vi "Promote Glue Routines.vi"(8 "error in (no error)":errorcluster, 11 "Assembly Run in":refnum<class "Assembly Run.lvclass">) -> (0 "error out":errorcluster, 3 "Assembly Run out":refnum<class "Assembly Run.lvclass">)   [LabVIEW 2021, in "Assembly Run.lvclass"]
uses:
  Assembly Run.lvclass
  Assembly Run.lvclass/Assembly Run.ctl
  Routine/Settings.ctl
  Routine/Routine Enum.ctl
  Workspace/Fixture Enum.ctl
  Workspace/Fixture.lvclass
  Routine/Routine.lvclass
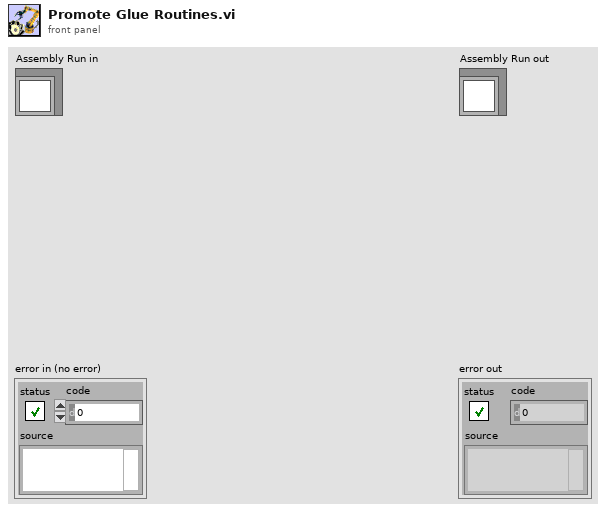
[diagram p1: front panel]
types:
  T1 = typedef "Fixture.lvclass/Fixture Enum.ctl" = enum16{"Assembly Tray", "Syringe Space", "Component", "Pick Up Tool", "Current Position"}
  T2 = typedef "Routine.lvclass/Routine Enum.ctl" = enum16{"Primary Pick Up", "Secondary Pick Up", "Put Down All", "Secure Syringe", "Release Syringe", "Dispense on Plate", "Dispense on Sensor", "Pick Up All", "Put Down Secondary", "Dispense on Kapton"}
  T3 = typedef "Routine.lvclass/Settings.ctl" = enum16{"Default", "Custom"}
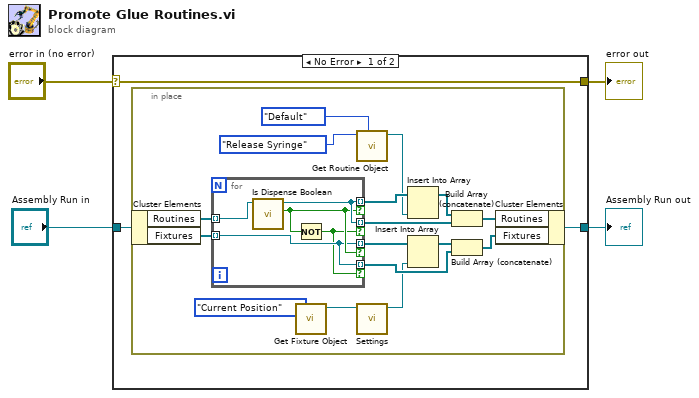
[diagram p0: block diagram]
diagram:
  n1 = case shown="No Error" "error in (no error)" {
    selector: "error in (no error)" -> [w7 w30]
    tunnel: [w7 w30] -> w3
    tunnel: [w5 w29] -> w2
    tunnel: "Assembly Run in" -> [w6 w29]
    frame No Error {
      n2 = in-place {
        n3 = in-place-cluster #1(w6) -> ("Routines"=w21:refnum<class "Routine.lvclass">[], "Fixtures"=w20:refnum<class "Fixture.lvclass">[])
        n4 = for {
          tunnel: w21 -> [w28] mode=indexing
          tunnel: w20 -> [w25] mode=indexing
          tunnel: [w27] -> w16 mode=indexing if=w26
          tunnel: [w27] -> w23 mode=indexing if=w24
          tunnel: [w25] -> w11 mode=indexing if=w26
          tunnel: [w25] -> w22 mode=indexing if=w24
          n5 = call-dynamic "Is Dispense Boolean.vi"("Routine in"=w28) -> ("Is Dispense?"=w26:bool, "Routine out"=w27:refnum<class "Routine.lvclass">)  [unwired: 8 in, 1 out]
          n6 = Not(x=w26) -> (.not. x?=w24:bool)
        }
        n7 = call "Get Fixture Object.vi"("Fixture"=Fixture_Enum."Current Position") -> ("Workspace.lvclass"=w9:refnum<class "Fixture.lvclass">)  [unwired: 8 in, 2 out]
        n8 = call "Get Routine Object.vi"("Settings"=Settings."Default", "Routine"=Routine_Enum."Release Syringe") -> ("Routine out"=w15:refnum<class "Routine.lvclass">)  [unwired: 8 in, 1 out]
        n9 = call-dynamic "Settings.vi"("Workspace in"=w9) -> ("Workspace out"=w8:refnum<class "Fixture.lvclass">)  [unwired: 9 in, 1 out]
        n10 = Insert Into Array(array=w16, new element=w15) -> (w14:refnum<class "Routine.lvclass">[])  [unwired: 1 in]
        n11 = Insert Into Array(array=w11, new element=w8) -> (w12:refnum<class "Fixture.lvclass">[])  [unwired: 1 in]
        n12 = Build Array (concatenate)(w14, w23) -> (w13:refnum<class "Routine.lvclass">[])
        n13 = Build Array (concatenate)(w12, w22) -> (w19:refnum<class "Fixture.lvclass">[])
        n14 = in-place-cluster #1("Routines"=w13, "Fixtures"=w19) -> (w5:refnum<class "Assembly Run.lvclass">)
      }
    }
    frame Error {
    }
  }
  "error out" <- w3
  "Assembly Run out" <- w2
